vi "PRL STR Convert Number to String.vi"(10 "Precision":i32, 11 "Number":dbl) -> (3 "Number String":string)   [LabVIEW 2013, in "PMU Recorder Light.lvlib"]
uses:
  PMU Recorder Light.lvlib
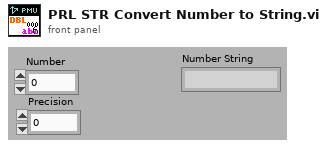
[diagram p1: front panel]
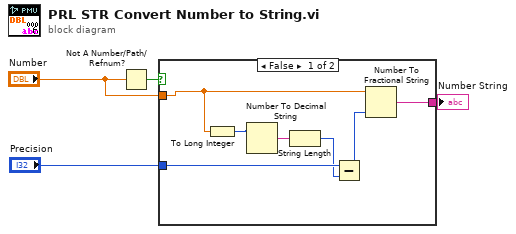
[diagram p0: block diagram]
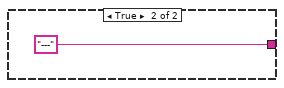
[diagram p2: hidden frame]
diagram:
  n1 = Not A Number/Path/Refnum?(number/path/refnum="Number") -> (NaN/Path/Refnum?=w4:bool)
  n2 = case shown="False" w4 {
    tunnel: [w11 "---"] -> w1
    tunnel: "Precision" -> [w7 _]
    tunnel: "Number" -> [w10 _]
    frame False {
      n3 = To Long Integer(number=w10) -> (32bit integer=w9:i32)
      n4 = Number To Decimal String(number=w9) -> (decimal integer string=w8:string)  [unwired: 1 in]
      n5 = String Length(string=w8) -> (length=w6:i32)
      n6 = Subtract(x=w7, y=w6) -> (x-y=w5:i32)
      n7 = Number To Fractional String(number=w10, precision (6)=w5) -> (F-format string=w11:string)  [unwired: 2 in]
    }
    frame True {
    }
  }
  "Number String" <- w1
